vi "test split quoted string.vi"() -> (2 "pass":bool)   [LabVIEW 2019, in "ANODE Tests.lvlib"]
uses:
  ANODE Tests.lvlib
panel:
  out "five":bool
  out "four":bool
  out "three":bool
  out "two":bool
  out "one":bool
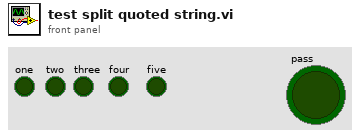
[diagram p1: front panel]
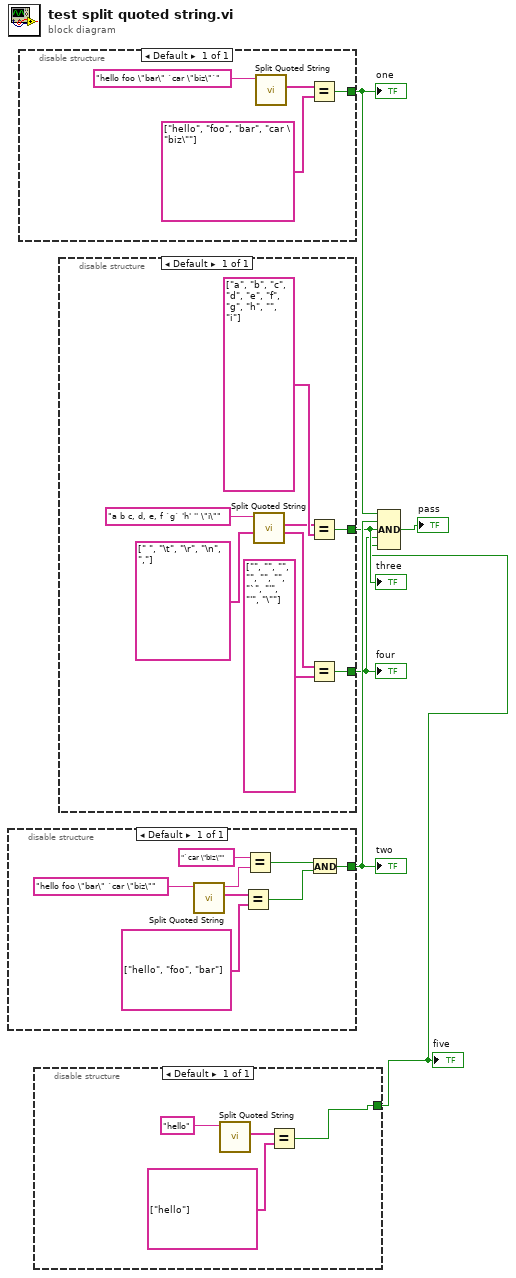
[diagram p0: block diagram]
diagram:
  n1 = disable-structure shown="Default" {
    disable-tunnel: [w8] -> w5
    frame Enabled {
      n2 = call "Split Quoted String.vi"("quoted string"="hello foo \"bar\" `car \"biz\"") -> ("elements"=w11:string[], "remaining string"=w10:string)  [unwired: 8 in, 1 out]
      n3 = Equal?(x=w11, y=string[] ["hello", "foo", "bar"] ("elements")) -> (x = y?=w12:bool)
      n4 = Equal?(x="`car \"biz\"" ("String"), y=w10) -> (x = y?=w7:bool)
      n5 = And(x=w7, y=w12) -> (x .and. y?=w8:bool)
    }
  }
  "two" <- w5
  n6 = disable-structure shown="Default" {
    disable-tunnel: [w16] -> w6
    frame Enabled {
      n7 = call "Split Quoted String.vi"("quoted string"="hello foo \"bar\" `car \"biz\"`") -> ("elements"=w15:string[])  [unwired: 8 in, 2 out]
      n8 = Equal?(x=w15, y=string[] ["hello", "foo", "bar", "car \"biz\""] ("elements")) -> (x = y?=w16:bool)
    }
  }
  "one" <- w6
  n9 = disable-structure shown="Default" {
    disable-tunnel: [w19] -> w1
    frame Enabled {
      n10 = call "Split Quoted String.vi"("quoted string"="hello") -> ("elements"=w20:string[])  [unwired: 8 in, 2 out]
      n11 = Equal?(x=w20, y=string[] ["hello"] ("elements")) -> (x = y?=w19:bool)
    }
  }
  "five" <- w1
  n12 = disable-structure shown="Default" {
    disable-tunnel: [w29] -> w3
    disable-tunnel: [w25] -> w2
    frame Enabled {
      n13 = call "Split Quoted String.vi"("delimiters (\\s,\\t,\\r,\\n)"=string[] [" ", "\t", "\r", "\n", ","] ("delimiters (\\s,\\t,\\r,\\n)"), "quoted string"="a b c, d, e, f `g` 'h' '' \"i\"") -> ("quote type"=w23:string[], "elements"=w24:string[])  [unwired: 7 in, 1 out]
      n14 = Equal?(x=w24, y=string[] ["a", "b", "c", "d", "e", "f", "g", "h", "", "i"] ("elements")) -> (x = y?=w29:bool)
      n15 = Equal?(x=w23, y=string[] ["", "", "", "", "", "", "`", "'", "'", "\""] ("quote type")) -> (x = y?=w25:bool)
    }
  }
  "three" <- w3
  "four" <- w2
  n16 = Compound Arithmetic op=AND(w6, w5, w3, w2, w1) -> (→"pass":bool)
